vi "Aperture.vi"() -> ()   [LabVIEW 2020]
uses:
  <instrlib>/Keithley 2600 Series/Public/Configure/Source/Configure Source (Range).vi
  <instrlib>/Keithley 2600 Series/Public/Configure/Source/Configure Source (Level).vi
  <instrlib>/Keithley 2600 Series/Public/Configure/Source/Configure Source (Limit).vi
  <instrlib>/Keithley 2600 Series/Keithley 2600 Series.lvlib
panel:
  in  "Current Limit (0.1 A)":dbl=0.1
  in  "Voltage Level (1 V)":dbl=1.0
  in  "Source Function (1: Voltage)":i32(ring)=1 items=["Voltage"=1]
  in  "Source Measure Unit Channel (0: Channel A)":i32(ring) items=["Channel A", "Channel B"]
  in  "VISA resource name":refnum<visa-resource-name>
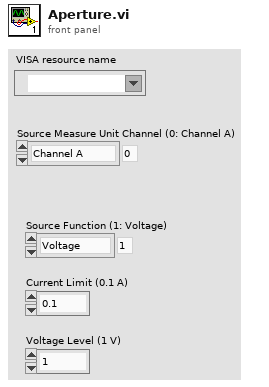
[diagram p1: front panel]
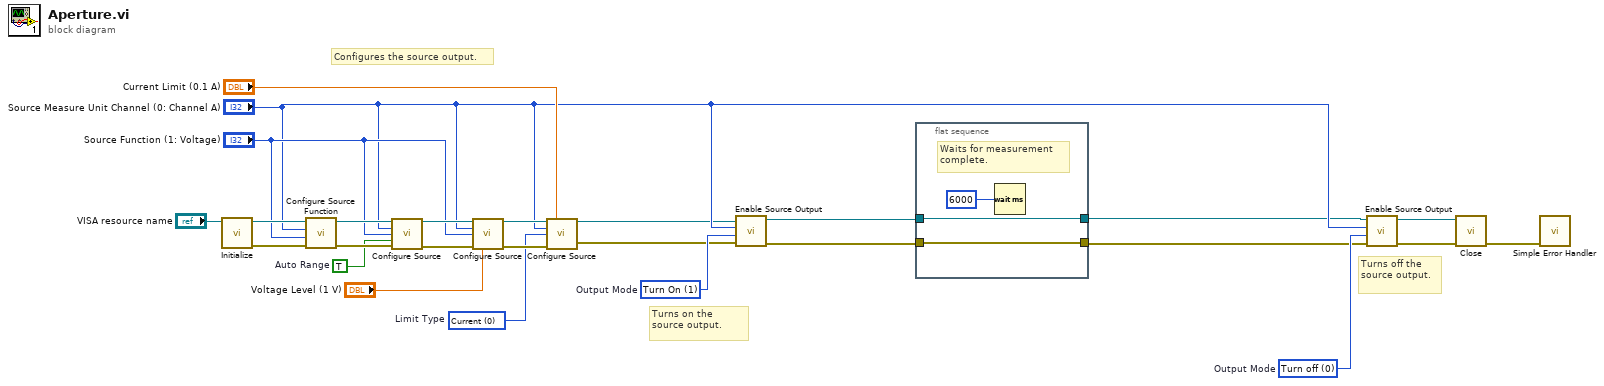
[diagram p0: block diagram]
diagram:
  w7 = 0 items=["Current", "Voltage", "Power"]  # Limit Type
  w12 = 0 items=["Turn off", "Turn On", "High-Z"]  # Output Mode
  w13 = 1 items=["Turn off", "Turn On", "High-Z"]  # Output Mode
  w19 = TRUE  # Auto Range
  # "Turns on the source output."
  # "Configures the source output."
  # "Turns off the source output."
  n1 = call <instrlib>:"Initialize.vi"("VISA resource name"="VISA resource name") -> ("error out"=w24:errorcluster, "VISA resource name out"=w25:refnum<visa-resource-name>)  [unwired: 9 in]
  n2 = call <instrlib>:"Configure Source Function.vi"("error in (no error)"=w24, "Source Function (1: Voltage)"="Source Function (1: Voltage)", "Source Measure Unit Channel (0: Channel A)"="Source Measure Unit Channel (0: Channel A)", "VISA resource name"=w25) -> ("error out"=w22:errorcluster, "VISA resource name out"=w23:refnum<visa-resource-name>)  [unwired: 6 in]
  n3 = call-poly <instrlib>:"Configure Source.vi"("VISA resource name"=w23, "Source Measure Unit Channel (0: Channel A)"="Source Measure Unit Channel (0: Channel A)", "Range Type (1: Voltage)"="Source Function (1: Voltage)", "Auto Range (T: Enable)"=w19, "error in (no error)"=w22) -> ("VISA resource name out"=w21:refnum<visa-resource-name>, "error out"=w20:errorcluster)  [unwired: 9 in]
  n4 = call-poly <instrlib>:"Configure Source.vi"("VISA resource name"=w21, "Source Measure Unit Channel (0: Channel A)"="Source Measure Unit Channel (0: Channel A)", "Level Type (1: Voltage)"="Source Function (1: Voltage)", "error in (no error)"=w20, "Voltage Level (0 V)"="Voltage Level (1 V)") -> ("VISA resource name out"=w17:refnum<visa-resource-name>, "error out"=w16:errorcluster)  [unwired: 9 in]
  n5 = call-poly <instrlib>:"Configure Source.vi"("VISA resource name"=w17, "Current Limit (0.1 A)"="Current Limit (0.1 A)", "Source Measure Unit Channel (0: Channel A)"="Source Measure Unit Channel (0: Channel A)", "Limit Type (1: Voltage)"=w7, "error in (no error)"=w16) -> ("VISA resource name out"=w6:refnum<visa-resource-name>, "error out"=w5:errorcluster)  [unwired: 9 in]
  n6 = call <instrlib>:"Enable Source Output.vi"("error in (no error)"=w5, "Output Mode (0: Turn off)"=w13, "Source Measure Unit Channel (0: Channel A)"="Source Measure Unit Channel (0: Channel A)", "VISA resource name"=w6) -> ("error out"=w3:errorcluster, "VISA resource name out"=w4:refnum<visa-resource-name>)  [unwired: 6 in]
  n7 = flat-sequence {
    tunnel: w4 -> [w27]
    tunnel: w3 -> [w28]
    tunnel: [w28] -> w1
    tunnel: [w27] -> w2
    frame #0 {
      # "Waits for measurement complete."
      n8 = Wait (ms)(milliseconds to wait=6000) -> ()  [unwired: 1 out]
    }
  }
  n9 = call <instrlib>:"Enable Source Output.vi"("error in (no error)"=w1, "Output Mode (0: Turn off)"=w12, "Source Measure Unit Channel (0: Channel A)"="Source Measure Unit Channel (0: Channel A)", "VISA resource name"=w2) -> ("error out"=w9:errorcluster, "VISA resource name out"=w10:refnum<visa-resource-name>)  [unwired: 6 in]
  n10 = call <instrlib>:"Close.vi"("error in (no error)"=w9, "VISA resource name"=w10) -> ("error out"=w8:errorcluster)  [unwired: 9 in]
  n11 = call <vilib>:"Simple Error Handler.vi"("error in (no error)"=w8) -> ()  [unwired: 4 in, 5 out]
